vi "EMG_State_Machine.vi"(0 "VISA Refnum in":refnum<visa-resource-name>, 1 "Positions":T4, 2 "EMG signal max amplitude (V)":dbl, 5 "EMG Control":T2(ring), 7 "Mode in":enum16{" M3", " M2", " M1"}(ring), 9 "System calibrated?":bool, 11 "error in (no error)":errorcluster, 12 "New Hand Positions in":T1(array[cluster]), 13 "EMG signal mean amplitude (V)":dbl) -> (3 "Mode":enum16{" M3", " M2", " M1"}(ring), 4 "VISA Refnum out":refnum<visa-resource-name>, 6 "New Hand Positions out":T1(array[cluster]), 8 "Mode out":enum16{" M3", " M2", " M1"}(ring), 10 "Mover4 Data":T3, 15 "error out":errorcluster)   [LabVIEW 2015]
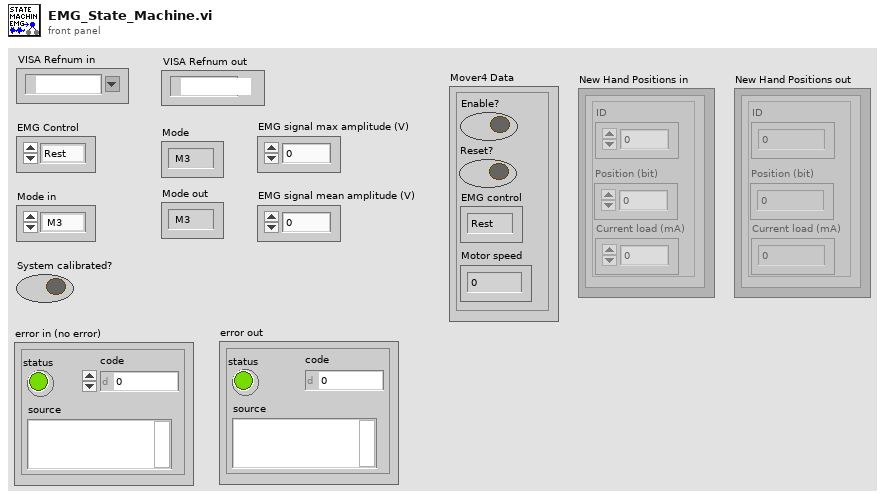
[diagram p1: front panel]
types:
  T1 = cluster{"ID":u16, "Position (bit)":u16, "Current load (mA)":u16}[]
  T2 = enum16{"Rest", "Triceps hardly contracted", "Triceps contracted", "Biceps hardly contracted", "Biceps contracted", "Change mode"}
  T3 = cluster{"Enable?":bool, "Reset?":bool, "EMG control":enum16{"Rest", "Biceps contracted", "Triceps contracted"}, "Motor speed":u8}
  T4 = cluster{"ID":u16, "Position (bit)":u16, "Current load (mA)":u16}
  T5 = enum16{"Rest", "Triceps hardly contracted M3", "Triceps hardly contracted M2", "Triceps hardly contracted M1", "Triceps contracted M3", "Triceps contracted M2", "Triceps contracted M1", "Biceps hardly contracted M3", "Biceps hardly contracted M2", "Biceps hardly contracted M1", "Biceps contracted M3", "Biceps contracted M2", "Biceps contracted M1", "Change mode"}
  T6 = enum16{"Biceps contracted", "Triceps contracted"}
  T7 = enum16{"Biceps contracted M3", "Biceps contracted", "Triceps contracted M3", "Triceps contracted"}
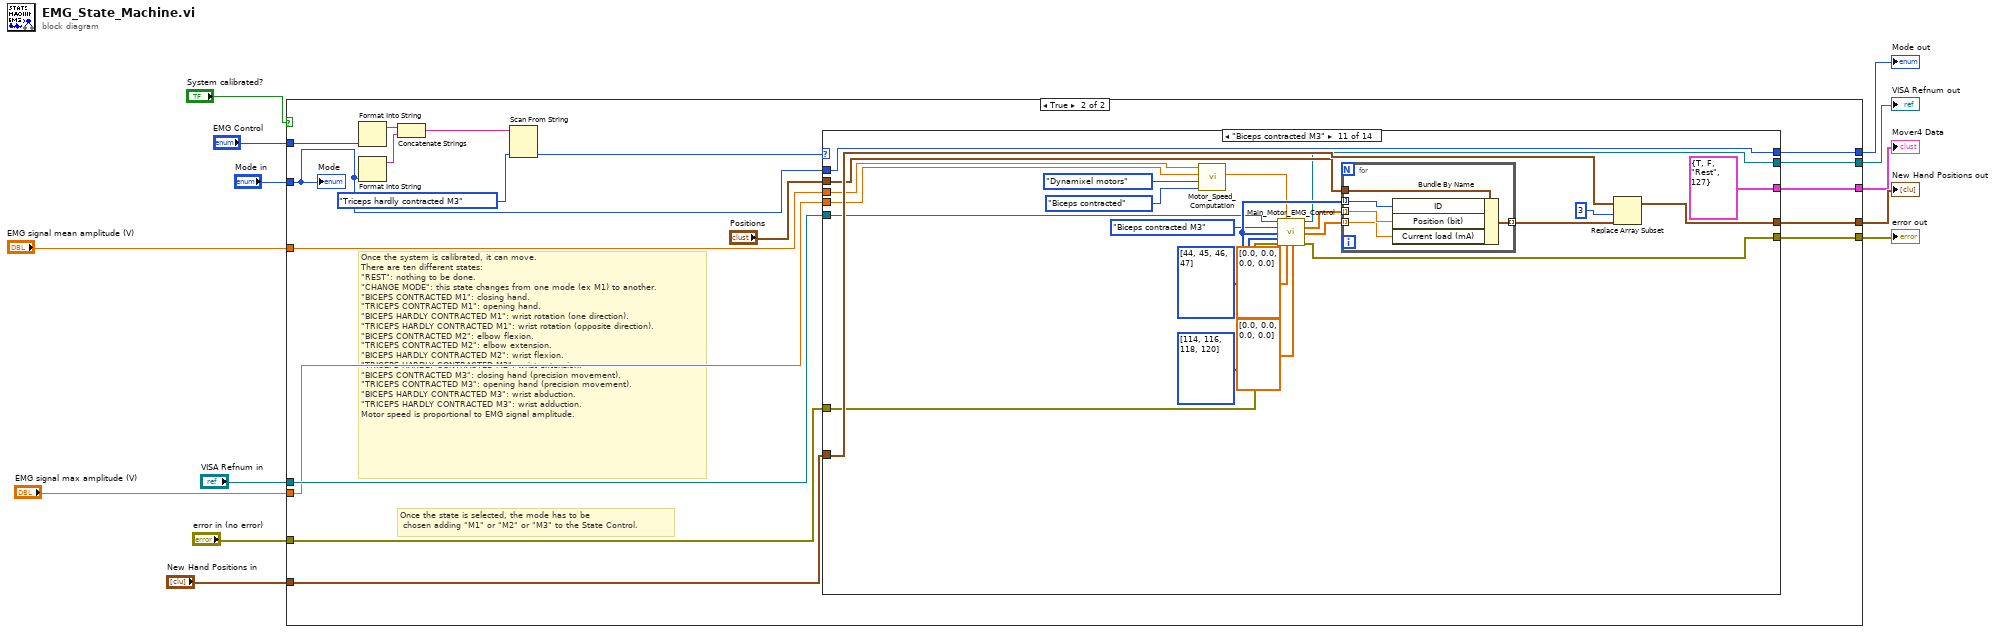
[diagram p0: block diagram]
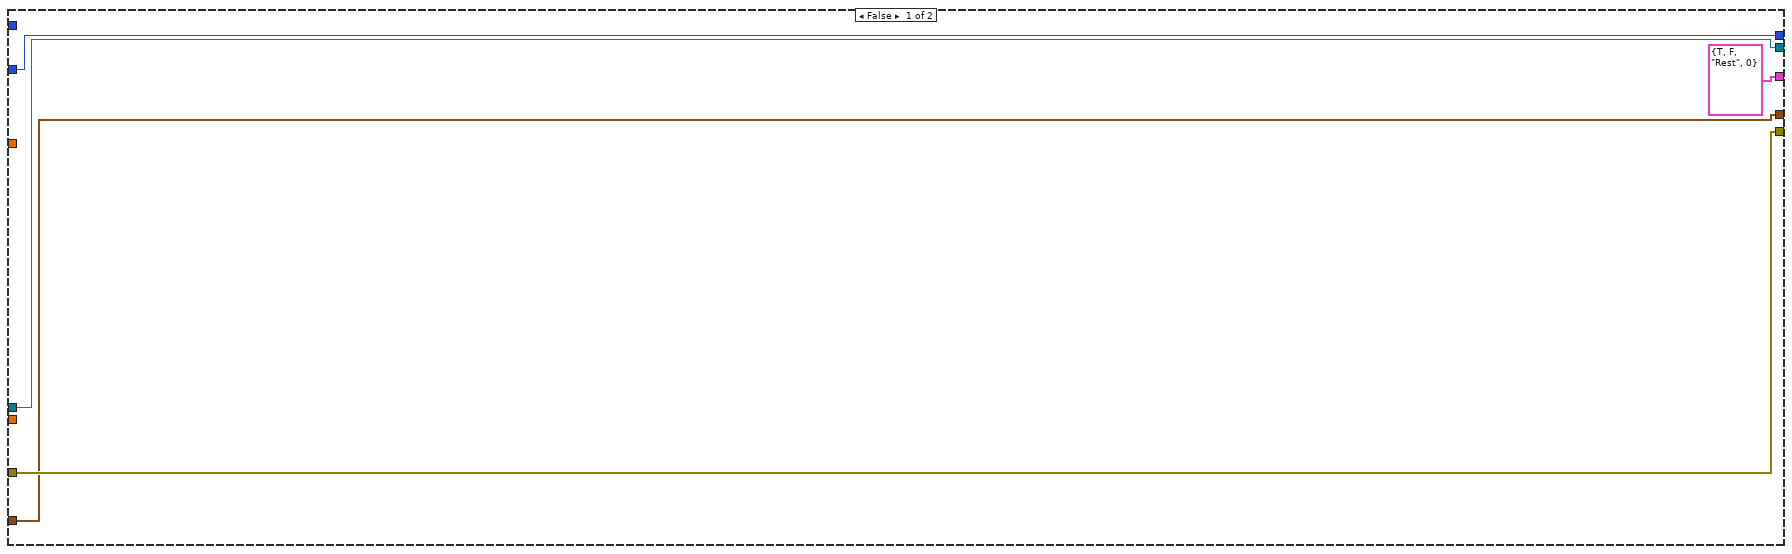
[diagram p2: hidden frame]
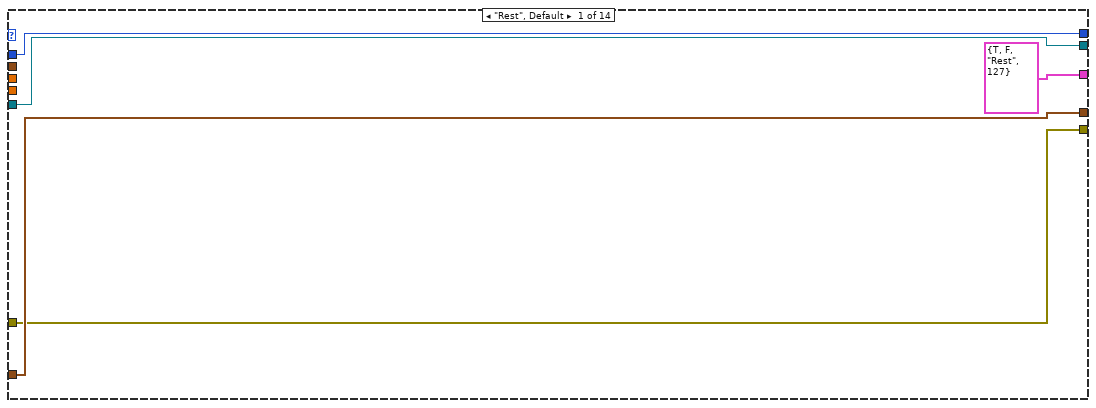
[diagram p3: hidden frame]
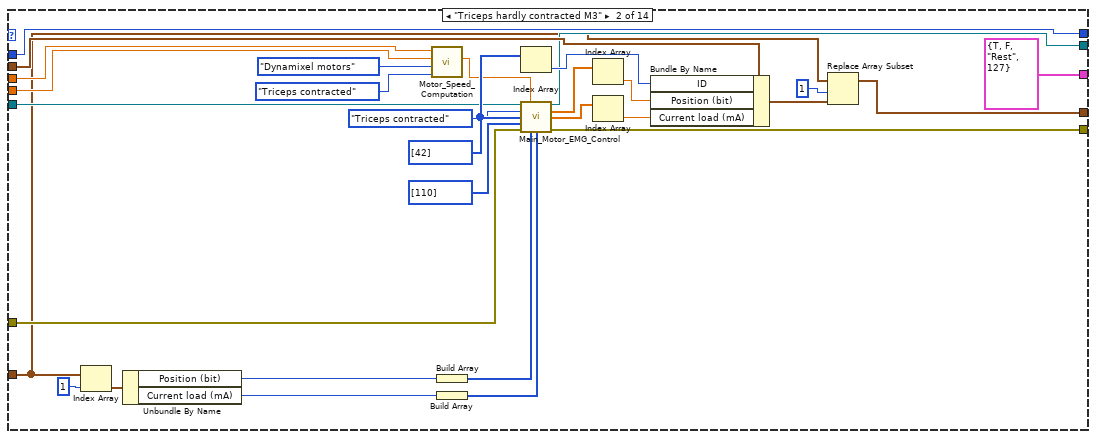
[diagram p4: hidden frame]
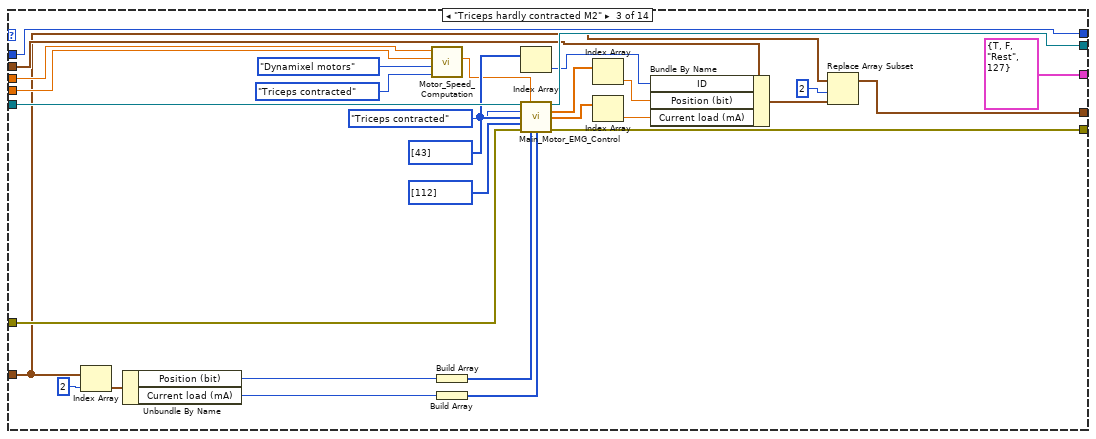
[diagram p5: hidden frame]
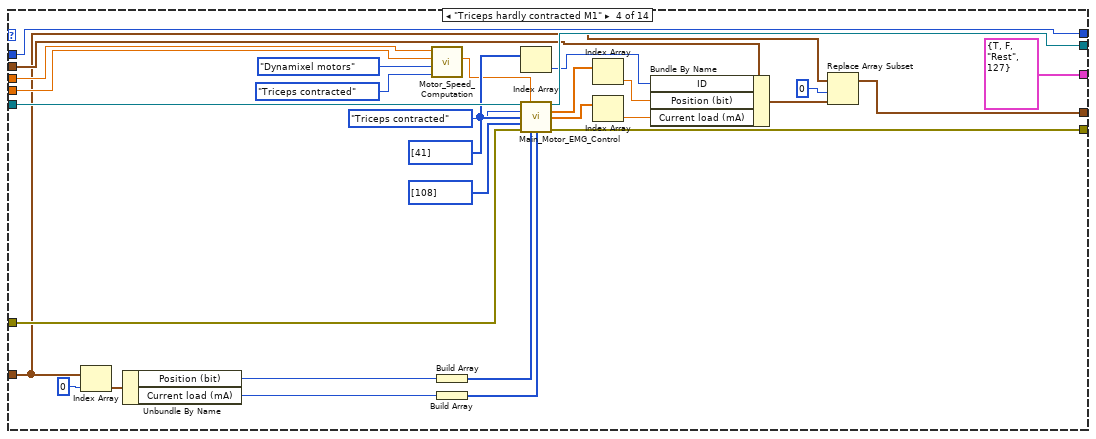
[diagram p6: hidden frame]
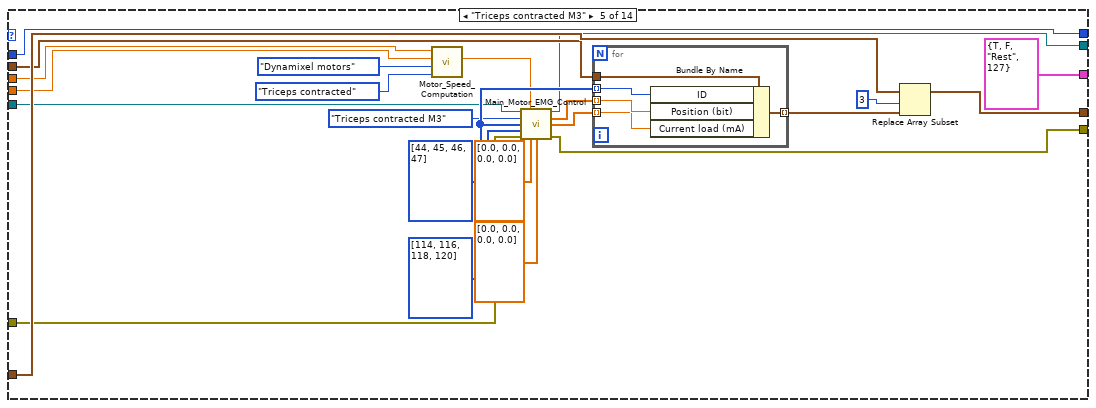
[diagram p7: hidden frame]
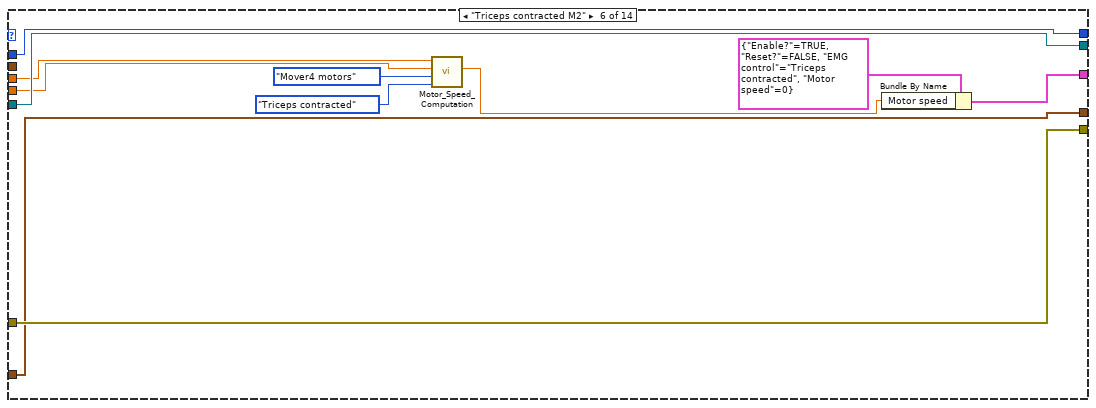
[diagram p8: hidden frame]
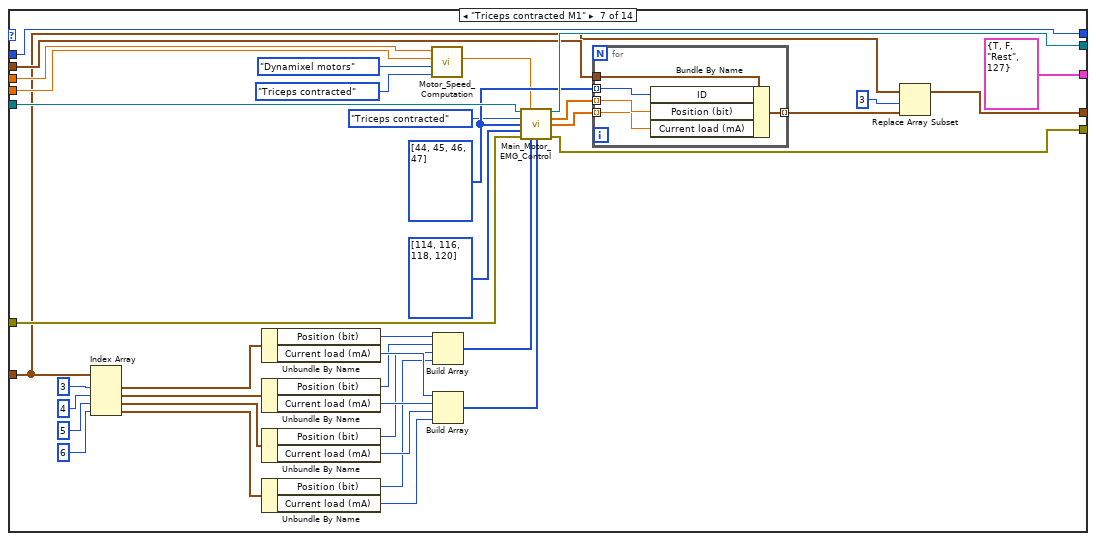
[diagram p9: hidden frame]
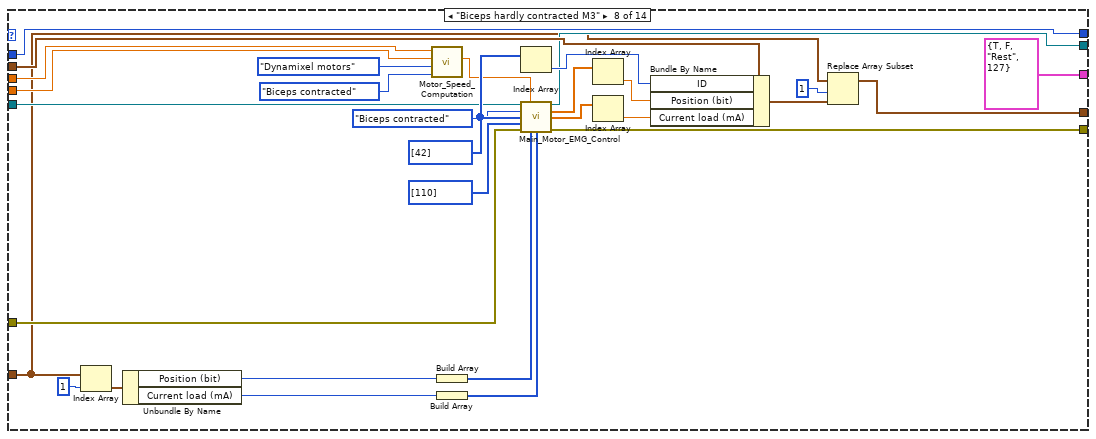
[diagram p10: hidden frame]
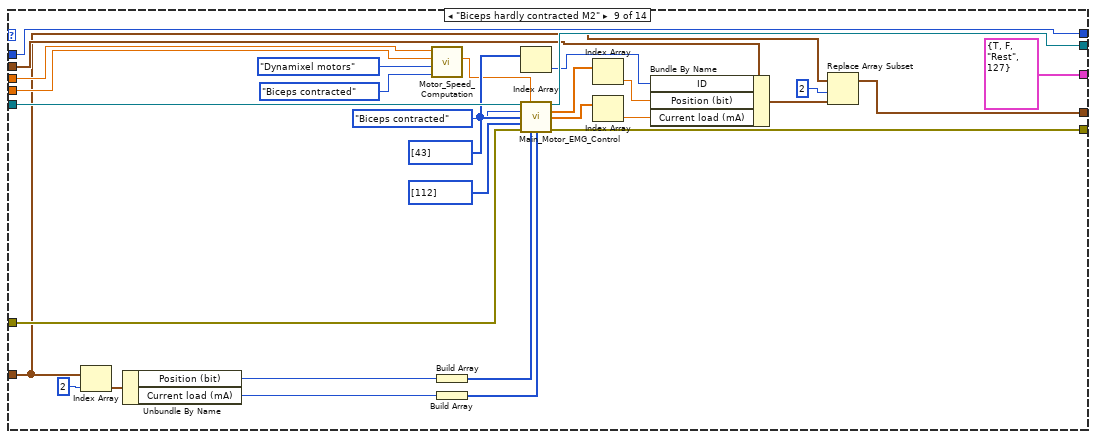
[diagram p11: hidden frame]
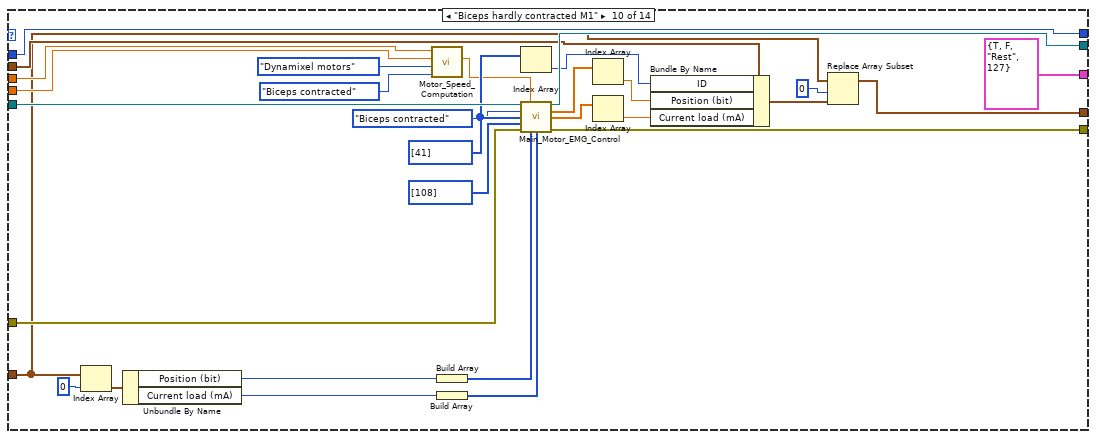
[diagram p12: hidden frame]
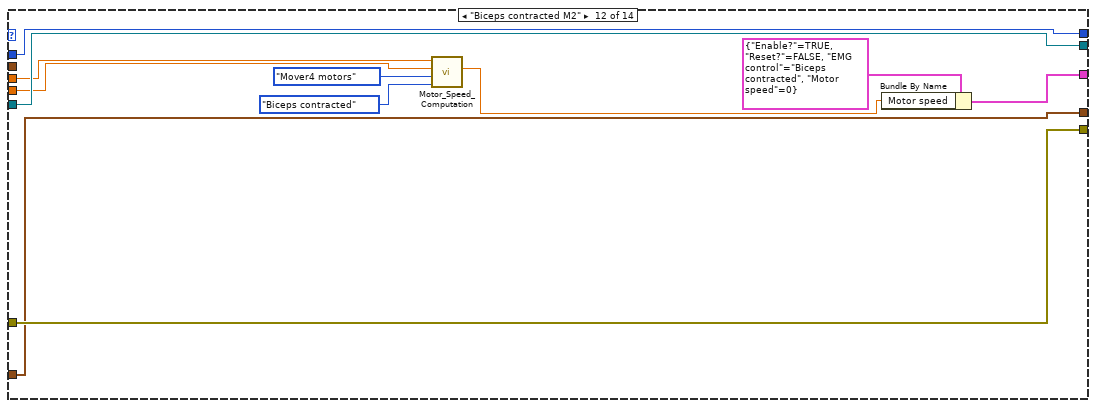
[diagram p13: hidden frame]
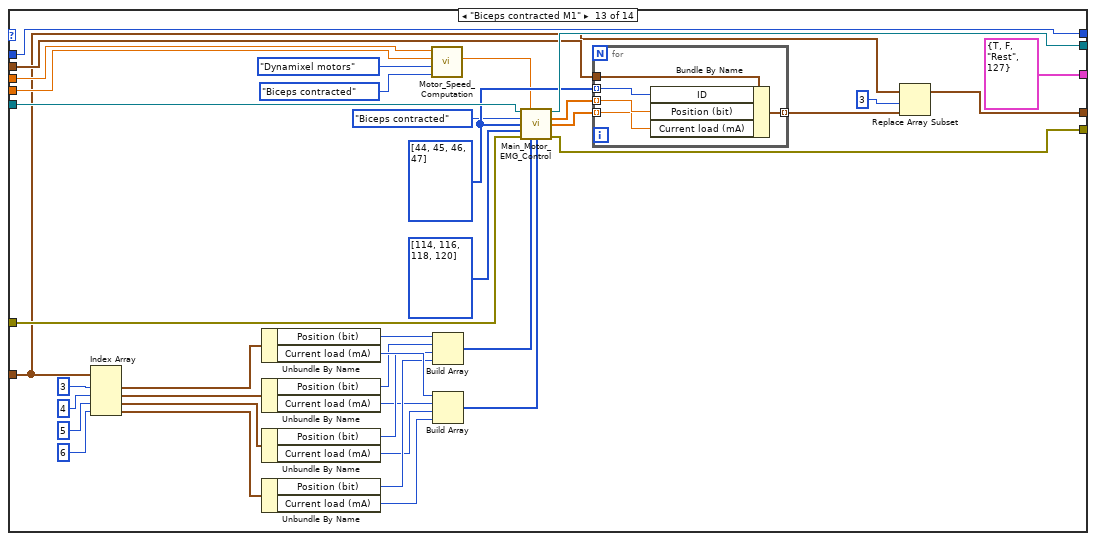
[diagram p14: hidden frame]
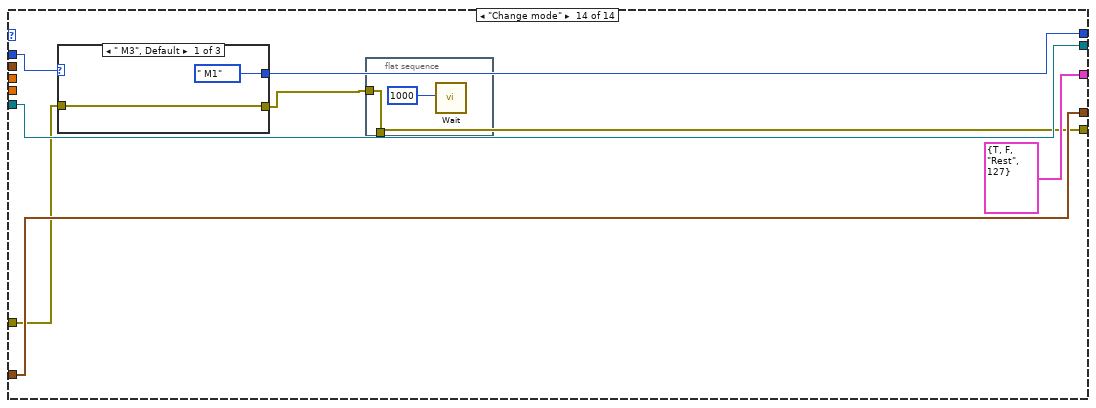
[diagram p15: hidden frame]
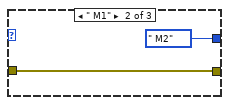
[diagram p16: hidden frame]
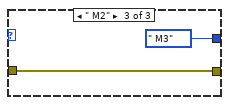
[diagram p17: hidden frame]
diagram:
  n1 = case shown="True" "System calibrated?" {
    tunnel: "VISA Refnum in" -> [w17 w34]
    tunnel: [w15 w23] -> w6
    tunnel: "EMG Control" -> [_ w26]
    tunnel: "error in (no error)" -> [w16 w35]
    tunnel: "Mode in" -> [w18 w27]
    tunnel: [w17 w24] -> w10
    tunnel: [w16 w22] -> w11
    tunnel: [w18 w25] -> w12
    tunnel: "New Hand Positions in" -> [w15 w36]
    tunnel: [T3 {"Enable?"=TRUE, "Reset?"=FALSE, "EMG control"=enum."Rest", "Motor speed"=0} ("data in") w19] -> w1
    tunnel: "EMG signal mean amplitude (V)" -> [_ w21]
    tunnel: "EMG signal max amplitude (V)" -> [_ w20]
    frame False {
    }
    frame True {
      # "Once the state is selected, the mode has to be\n chosen adding \"M1\" or \"M2\" or \"M3\" to the State Control."
      # "Once the system is calibrated, it can move.\nThere are ten different states:\n\"REST\": nothing to be done.\n\"CHANGE MODE\": this state changes from one mode (ex M1) to another.\n\"BICEPS CONTRACTED M1\": closing hand.\n\"TRICEPS CONTRACTED M1\": opening hand.\n\"BICEPS HARDLY CONTRACTED M1\": wrist rotation (one direction).\n\"TRICEPS HARDLY CONTRACTED M1\": wrist rotation (opposite direction).\n\"BICEPS CONTRACTED M2\": elbow flexion.\n\"TRICEPS CONTRACTED M2\": elbow extension.\n\"BICEPS HARDLY CONTRACTED M2\": wrist flexion.\n\"TRICEPS HARDLY CONTRACTED M2\": wrist extension.\n\"BICEPS CONTRACTED M3\": closing hand (precision movement).\n\"TRICEPS CONTRACTED M3\": opening hand (precision movement).\n\"BICEPS HARDLY CONTRACTED M3\": wrist abduction.\n\"TRICEPS HARDLY CONTRACTED M3\": wrist adduction.\nMotor speed is proportional to EMG signal amplitude."
      n2 = Format Into String(w26) -> (resulting string=w32:string)  [unwired: 3 in, 1 out]
      n3 = Format Into String(w27) -> (resulting string=w29:string)  [unwired: 3 in, 1 out]
      n4 = Concatenate Strings(w32, w29) -> (w30:string)
      n5 = Scan From String(input string=w30, default 1=T5."Triceps hardly contracted M3") -> (output 1=w28:T5)  [unwired: 3 in, 3 out]
      n6 = case shown="\"Biceps contracted M3\"" w28 {
        tunnel: w34 -> [w41 w61 w99 w127 w145 w170 w205 w233 w270 w303 w314 w343 w382 w395]
        tunnel: w35 -> [w38 w60 w100 w128 w144 w169 w206 w232 w271 w302 w317 w342 w381 w390]
        tunnel: [w41 w59 w98 w130 w141 w170 w208 w231 w273 w301 w315 w343 w380 w395] -> w24
        tunnel: [w38 w58 w97 w129 w143 w169 w207 w230 w272 w300 w316 w342 w379 w388] -> w22
        tunnel: [w40 w56 w96 w126 w148 w168 w204 w235 w269 w299 w321 w341 w377 w392] -> w25
        tunnel: w27 -> [w40 w56 w96 w126 w148 w168 w204 w235 w269 w299 w321 w341 w377 w393]
        tunnel: w36 -> [w39 w44 w74 w108 w147 w167 w185 w217 w247 w277 w319 w340 w358 w394]
        tunnel: [w39 w57 w87 w120 w142 w167 w199 w229 w264 w294 w320 w340 w374 w394] -> w23
        tunnel: "Positions" -> [_ w62 w86 w116 w146 _ w203 w234 w260 w289 w318 _ w373 _]
        tunnel: [T3 {"Enable?"=TRUE, "Reset?"=FALSE, "EMG control"=enum."Rest", "Motor speed"=127} ("data in") T3 {"Enable?"=TRUE, "Reset?"=FALSE, "EMG control"=enum."Rest", "Motor speed"=127} ("data in") T3 {"Enable?"=TRUE, "Reset?"=FALSE, "EMG control"=enum."Rest", "Motor speed"=127} ("data in") T3 {"Enable?"=TRUE, "Reset?"=FALSE, "EMG control"=enum."Rest", "Motor speed"=127} ("data in") T3 {"Enable?"=TRUE, "Reset?"=FALSE, "EMG control"=enum."Rest", "Motor speed"=127} ("data in") w161 T3 {"Enable?"=TRUE, "Reset?"=FALSE, "EMG control"=enum."Rest", "Motor speed"=127} ("data in") T3 {"Enable?"=TRUE, "Reset?"=FALSE, "EMG control"=enum."Rest", "Motor speed"=127} ("data in") T3 {"Enable?"=TRUE, "Reset?"=FALSE, "EMG control"=enum."Rest", "Motor speed"=127} ("data in") T3 {"Enable?"=TRUE, "Reset?"=FALSE, "EMG control"=enum."Rest", "Motor speed"=127} ("data in") T3 {"Enable?"=TRUE, "Reset?"=FALSE, "EMG control"=enum."Rest", "Motor speed"=127} ("data in") w337 T3 {"Enable?"=TRUE, "Reset?"=FALSE, "EMG control"=enum."Rest", "Motor speed"=127} ("data in") T3 {"Enable?"=TRUE, "Reset?"=FALSE, "EMG control"=enum."Rest", "Motor speed"=127} ("data in")] -> w19
        tunnel: w21 -> [_ w51 w80 w111 w137 w164 w192 w224 w254 w284 w309 w336 w365 _]
        tunnel: w20 -> [_ w50 w81 w112 w136 w163 w191 w223 w253 w283 w308 w335 w366 _]
        frame "Rest", Default {
        }
        frame "Triceps hardly contracted M3" {
          w70 = i32[] [42] ("ID motors")
          n7 = Index Array(array=w44, index=1) -> (element=w47:T4)
          n8 = Unbundle By Name(w47) -> ("Position (bit)"=w46:u16, "Current load (mA)"=w45:u16)
          n9 = call "Motor_Speed_Computation.vi"("Contracted muscle"=T6."Triceps contracted", "Motor type"=enum16{"Mover4 motors", "Dynamixel motors"}."Dynamixel motors", "EMG signal max amplitude (V)"=w50, "EMG signal mean amplitude (V)"=w51) -> ("Motor speed (RPM or bit)"=w52:dbl)  [unwired: 7 in]
          n10 = Build Array(w46) -> (w43:u16[])
          n11 = Build Array(w45) -> (w42:u16[])
          n12 = Index Array(array=w70) -> (element=w69:i32)  [unwired: 1 in]
          n13 = call "Main_Motor_EMG_Control.vi"("VISA Refnum in"=w61, "Motor speed"=w52, "EMG control"=T7."Triceps contracted", "ID motors"=w70, "Address current load"=i32[] [110] ("ID motors"), "error in (no error)"=w60, "Old positions"=w43, "Old Current (mA)"=w42) -> ("VISA Refnum out"=w59:refnum<visa-resource-name>, "Actual positions"=w68:dbl[], "Current (mA)"=w66:dbl[], "error out"=w58:errorcluster)  [unwired: 4 in]
          n14 = Index Array(array=w68) -> (element=w67:dbl)  [unwired: 1 in]
          n15 = Index Array(array=w66) -> (element=w65:dbl)  [unwired: 1 in]
          n16 = Bundle By Name(cluster=w62, "ID"=w69, "Position (bit)"=w67, "Current load (mA)"=w65) -> (w64:T4)
          n17 = Replace Array Subset(array=w44, new element=w64, index=1) -> (w57:T1)
        }
        frame "Triceps hardly contracted M2" {
          w95 = i32[] [43] ("ID motors")
          n18 = Index Array(array=w74, index=2) -> (element=w77:T4)
          n19 = Unbundle By Name(w77) -> ("Position (bit)"=w76:u16, "Current load (mA)"=w75:u16)
          n20 = call "Motor_Speed_Computation.vi"("Contracted muscle"=T6."Triceps contracted", "Motor type"=enum16{"Mover4 motors", "Dynamixel motors"}."Dynamixel motors", "EMG signal max amplitude (V)"=w81, "EMG signal mean amplitude (V)"=w80) -> ("Motor speed (RPM or bit)"=w82:dbl)  [unwired: 7 in]
          n21 = Build Array(w76) -> (w73:u16[])
          n22 = Build Array(w75) -> (w72:u16[])
          n23 = Index Array(array=w95) -> (element=w94:i32)  [unwired: 1 in]
          n24 = call "Main_Motor_EMG_Control.vi"("VISA Refnum in"=w99, "Motor speed"=w82, "EMG control"=T7."Triceps contracted", "ID motors"=w95, "Address current load"=i32[] [112] ("ID motors"), "error in (no error)"=w100, "Old positions"=w73, "Old Current (mA)"=w72) -> ("VISA Refnum out"=w98:refnum<visa-resource-name>, "Actual positions"=w93:dbl[], "Current (mA)"=w91:dbl[], "error out"=w97:errorcluster)  [unwired: 4 in]
          n25 = Index Array(array=w93) -> (element=w92:dbl)  [unwired: 1 in]
          n26 = Index Array(array=w91) -> (element=w90:dbl)  [unwired: 1 in]
          n27 = Bundle By Name(cluster=w86, "ID"=w94, "Position (bit)"=w92, "Current load (mA)"=w90) -> (w89:T4)
          n28 = Replace Array Subset(array=w74, new element=w89, index=2) -> (w87:T1)
        }
        frame "Triceps hardly contracted M1" {
          w119 = i32[] [41] ("ID motors")
          n29 = Index Array(array=w108, index=0) -> (element=w106:T4)
          n30 = Unbundle By Name(w106) -> ("Position (bit)"=w105:u16, "Current load (mA)"=w103:u16)
          n31 = call "Motor_Speed_Computation.vi"("Contracted muscle"=T6."Triceps contracted", "Motor type"=enum16{"Mover4 motors", "Dynamixel motors"}."Dynamixel motors", "EMG signal max amplitude (V)"=w112, "EMG signal mean amplitude (V)"=w111) -> ("Motor speed (RPM or bit)"=w110:dbl)  [unwired: 7 in]
          n32 = Build Array(w105) -> (w104:u16[])
          n33 = Build Array(w103) -> (w102:u16[])
          n34 = Index Array(array=w119) -> (element=w125:i32)  [unwired: 1 in]
          n35 = call "Main_Motor_EMG_Control.vi"("VISA Refnum in"=w127, "Motor speed"=w110, "EMG control"=T7."Triceps contracted", "ID motors"=w119, "Address current load"=i32[] [108] ("ID motors"), "error in (no error)"=w128, "Old positions"=w104, "Old Current (mA)"=w102) -> ("VISA Refnum out"=w130:refnum<visa-resource-name>, "Actual positions"=w118:dbl[], "Current (mA)"=w117:dbl[], "error out"=w129:errorcluster)  [unwired: 4 in]
          n36 = Index Array(array=w118) -> (element=w124:dbl)  [unwired: 1 in]
          n37 = Index Array(array=w117) -> (element=w123:dbl)  [unwired: 1 in]
          n38 = Bundle By Name(cluster=w116, "ID"=w125, "Position (bit)"=w124, "Current load (mA)"=w123) -> (w122:T4)
          n39 = Replace Array Subset(array=w108, new element=w122, index=0) -> (w120:T1)
        }
        frame "Triceps contracted M3" {
          w151 = i32[] [44, 45, 46, 47] ("ID motors")
          n40 = call "Motor_Speed_Computation.vi"("Contracted muscle"=T6."Triceps contracted", "Motor type"=enum16{"Mover4 motors", "Dynamixel motors"}."Dynamixel motors", "EMG signal max amplitude (V)"=w136, "EMG signal mean amplitude (V)"=w137) -> ("Motor speed (RPM or bit)"=w135:dbl)  [unwired: 7 in]
          n41 = call "Main_Motor_EMG_Control.vi"("VISA Refnum in"=w145, "Motor speed"=w135, "EMG control"=T7."Triceps contracted M3", "ID motors"=w151, "Address current load"=i32[] [114, 116, 118, 120] ("ID motors"), "error in (no error)"=w144, "Old positions"=dbl[] [0.0, 0.0, 0.0, 0.0], "Old Current (mA)"=dbl[] [0.0, 0.0, 0.0, 0.0]) -> ("VISA Refnum out"=w141:refnum<visa-resource-name>, "Actual positions"=w150:dbl[], "Current (mA)"=w149:dbl[], "error out"=w143:errorcluster)  [unwired: 4 in]
          n42 = for {
            tunnel: w146 -> [w159]
            tunnel: w151 -> [w158] mode=indexing
            tunnel: w150 -> [w157] mode=indexing
            tunnel: w149 -> [w156] mode=indexing
            tunnel: [w155] -> w153 mode=indexing
            n43 = Bundle By Name(cluster=w159, "ID"=w158, "Position (bit)"=w157, "Current load (mA)"=w156) -> (w155:T4)
          }
          n44 = Replace Array Subset(array=w147, new element=w153, index=3) -> (w142:T1)
        }
        frame "Triceps contracted M2" {
          n45 = call "Motor_Speed_Computation.vi"("Contracted muscle"=T6."Triceps contracted", "Motor type"=enum16{"Mover4 motors", "Dynamixel motors"}."Mover4 motors", "EMG signal max amplitude (V)"=w163, "EMG signal mean amplitude (V)"=w164) -> ("Motor speed (RPM or bit)"=w162:dbl)  [unwired: 7 in]
          n46 = Bundle By Name(cluster=T3 {"Enable?"=TRUE, "Reset?"=FALSE, "EMG control"=enum."Triceps contracted", "Motor speed"=0} ("data in"), "Motor speed"=w162) -> (w161:T3)
        }
        frame "Triceps contracted M1" {
          w202 = i32[] [44, 45, 46, 47] ("ID motors")
          n47 = Index Array(array=w185, index #1=3 ("index"), index #2=4 ("index"), index #3=5 ("index"), index #4=6 ("index")) -> (element #1=w188:T4, element #2=w179:T4, element #3=w178:T4, element #4=w177:T4)
          n48 = Unbundle By Name(w188) -> ("Position (bit)"=w187:u16, "Current load (mA)"=w186:u16)
          n49 = Unbundle By Name(w179) -> ("Position (bit)"=w173:u16, "Current load (mA)"=w176:u16)
          n50 = Unbundle By Name(w178) -> ("Position (bit)"=w172:u16, "Current load (mA)"=w175:u16)
          n51 = Unbundle By Name(w177) -> ("Position (bit)"=w171:u16, "Current load (mA)"=w174:u16)
          n52 = call "Motor_Speed_Computation.vi"("Contracted muscle"=T6."Triceps contracted", "Motor type"=enum16{"Mover4 motors", "Dynamixel motors"}."Dynamixel motors", "EMG signal max amplitude (V)"=w191, "EMG signal mean amplitude (V)"=w192) -> ("Motor speed (RPM or bit)"=w190:dbl)  [unwired: 7 in]
          n53 = Build Array(w187, w173, w172, w171) -> (w181:u16[])
          n54 = Build Array(w186, w176, w175, w174) -> (w180:u16[])
          n55 = call "Main_Motor_EMG_Control.vi"("VISA Refnum in"=w205, "Motor speed"=w190, "EMG control"=T7."Triceps contracted", "ID motors"=w202, "Address current load"=i32[] [114, 116, 118, 120] ("ID motors"), "error in (no error)"=w206, "Old positions"=w181, "Old Current (mA)"=w180) -> ("VISA Refnum out"=w208:refnum<visa-resource-name>, "Actual positions"=w201:dbl[], "Current (mA)"=w200:dbl[], "error out"=w207:errorcluster)  [unwired: 4 in]
          n56 = for {
            tunnel: w203 -> [w214]
            tunnel: w202 -> [w213] mode=indexing
            tunnel: w201 -> [w212] mode=indexing
            tunnel: w200 -> [w211] mode=indexing
            tunnel: [w210] -> w198 mode=indexing
            n57 = Bundle By Name(cluster=w214, "ID"=w213, "Position (bit)"=w212, "Current load (mA)"=w211) -> (w210:T4)
          }
          n58 = Replace Array Subset(array=w185, new element=w198, index=3) -> (w199:T1)
        }
        frame "Biceps hardly contracted M3" {
          w243 = i32[] [42] ("ID motors")
          n59 = Index Array(array=w217, index=1) -> (element=w220:T4)
          n60 = Unbundle By Name(w220) -> ("Position (bit)"=w219:u16, "Current load (mA)"=w218:u16)
          n61 = call "Motor_Speed_Computation.vi"("Contracted muscle"=T6."Biceps contracted", "Motor type"=enum16{"Mover4 motors", "Dynamixel motors"}."Dynamixel motors", "EMG signal max amplitude (V)"=w223, "EMG signal mean amplitude (V)"=w224) -> ("Motor speed (RPM or bit)"=w222:dbl)  [unwired: 7 in]
          n62 = Build Array(w219) -> (w216:u16[])
          n63 = Build Array(w218) -> (w215:u16[])
          n64 = Index Array(array=w243) -> (element=w242:i32)  [unwired: 1 in]
          n65 = call "Main_Motor_EMG_Control.vi"("VISA Refnum in"=w233, "Motor speed"=w222, "EMG control"=T7."Biceps contracted", "ID motors"=w243, "Address current load"=i32[] [110] ("ID motors"), "error in (no error)"=w232, "Old positions"=w216, "Old Current (mA)"=w215) -> ("VISA Refnum out"=w231:refnum<visa-resource-name>, "Actual positions"=w241:dbl[], "Current (mA)"=w239:dbl[], "error out"=w230:errorcluster)  [unwired: 4 in]
          n66 = Index Array(array=w241) -> (element=w240:dbl)  [unwired: 1 in]
          n67 = Index Array(array=w239) -> (element=w238:dbl)  [unwired: 1 in]
          n68 = Bundle By Name(cluster=w234, "ID"=w242, "Position (bit)"=w240, "Current load (mA)"=w238) -> (w237:T4)
          n69 = Replace Array Subset(array=w217, new element=w237, index=1) -> (w229:T1)
        }
        frame "Biceps hardly contracted M2" {
          w263 = i32[] [43] ("ID motors")
          n70 = Index Array(array=w247, index=2) -> (element=w250:T4)
          n71 = Unbundle By Name(w250) -> ("Position (bit)"=w249:u16, "Current load (mA)"=w248:u16)
          n72 = call "Motor_Speed_Computation.vi"("Contracted muscle"=T6."Biceps contracted", "Motor type"=enum16{"Mover4 motors", "Dynamixel motors"}."Dynamixel motors", "EMG signal max amplitude (V)"=w253, "EMG signal mean amplitude (V)"=w254) -> ("Motor speed (RPM or bit)"=w252:dbl)  [unwired: 7 in]
          n73 = Build Array(w249) -> (w246:u16[])
          n74 = Build Array(w248) -> (w245:u16[])
          n75 = Index Array(array=w263) -> (element=w268:i32)  [unwired: 1 in]
          n76 = call "Main_Motor_EMG_Control.vi"("VISA Refnum in"=w270, "Motor speed"=w252, "EMG control"=T7."Biceps contracted", "ID motors"=w263, "Address current load"=i32[] [112] ("ID motors"), "error in (no error)"=w271, "Old positions"=w246, "Old Current (mA)"=w245) -> ("VISA Refnum out"=w273:refnum<visa-resource-name>, "Actual positions"=w262:dbl[], "Current (mA)"=w261:dbl[], "error out"=w272:errorcluster)  [unwired: 4 in]
          n77 = Index Array(array=w262) -> (element=w267:dbl)  [unwired: 1 in]
          n78 = Index Array(array=w261) -> (element=w259:dbl)  [unwired: 1 in]
          n79 = Bundle By Name(cluster=w260, "ID"=w268, "Position (bit)"=w267, "Current load (mA)"=w259) -> (w266:T4)
          n80 = Replace Array Subset(array=w247, new element=w266, index=2) -> (w264:T1)
        }
        frame "Biceps hardly contracted M1" {
          w293 = i32[] [41] ("ID motors")
          n81 = Index Array(array=w277, index=0) -> (element=w280:T4)
          n82 = Unbundle By Name(w280) -> ("Position (bit)"=w279:u16, "Current load (mA)"=w278:u16)
          n83 = call "Motor_Speed_Computation.vi"("Contracted muscle"=T6."Biceps contracted", "Motor type"=enum16{"Mover4 motors", "Dynamixel motors"}."Dynamixel motors", "EMG signal max amplitude (V)"=w283, "EMG signal mean amplitude (V)"=w284) -> ("Motor speed (RPM or bit)"=w282:dbl)  [unwired: 7 in]
          n84 = Build Array(w279) -> (w276:u16[])
          n85 = Build Array(w278) -> (w275:u16[])
          n86 = Index Array(array=w293) -> (element=w298:i32)  [unwired: 1 in]
          n87 = call "Main_Motor_EMG_Control.vi"("VISA Refnum in"=w303, "Motor speed"=w282, "EMG control"=T7."Biceps contracted", "ID motors"=w293, "Address current load"=i32[] [108] ("ID motors"), "error in (no error)"=w302, "Old positions"=w276, "Old Current (mA)"=w275) -> ("VISA Refnum out"=w301:refnum<visa-resource-name>, "Actual positions"=w292:dbl[], "Current (mA)"=w291:dbl[], "error out"=w300:errorcluster)  [unwired: 4 in]
          n88 = Index Array(array=w292) -> (element=w297:dbl)  [unwired: 1 in]
          n89 = Index Array(array=w291) -> (element=w290:dbl)  [unwired: 1 in]
          n90 = Bundle By Name(cluster=w289, "ID"=w298, "Position (bit)"=w297, "Current load (mA)"=w290) -> (w296:T4)
          n91 = Replace Array Subset(array=w277, new element=w296, index=0) -> (w294:T1)
        }
        frame "Biceps contracted M3" {
          w324 = i32[] [44, 45, 46, 47] ("ID motors")
          n92 = call "Motor_Speed_Computation.vi"("Contracted muscle"=T6."Biceps contracted", "Motor type"=enum16{"Mover4 motors", "Dynamixel motors"}."Dynamixel motors", "EMG signal max amplitude (V)"=w308, "EMG signal mean amplitude (V)"=w309) -> ("Motor speed (RPM or bit)"=w307:dbl)  [unwired: 7 in]
          n93 = call "Main_Motor_EMG_Control.vi"("VISA Refnum in"=w314, "Motor speed"=w307, "EMG control"=T7."Biceps contracted M3", "ID motors"=w324, "Address current load"=i32[] [114, 116, 118, 120] ("ID motors"), "error in (no error)"=w317, "Old positions"=dbl[] [0.0, 0.0, 0.0, 0.0], "Old Current (mA)"=dbl[] [0.0, 0.0, 0.0, 0.0]) -> ("VISA Refnum out"=w315:refnum<visa-resource-name>, "Actual positions"=w323:dbl[], "Current (mA)"=w322:dbl[], "error out"=w316:errorcluster)  [unwired: 4 in]
          n94 = for {
            tunnel: w318 -> [w332]
            tunnel: w324 -> [w331] mode=indexing
            tunnel: w323 -> [w330] mode=indexing
            tunnel: w322 -> [w329] mode=indexing
            tunnel: [w328] -> w326 mode=indexing
            n95 = Bundle By Name(cluster=w332, "ID"=w331, "Position (bit)"=w330, "Current load (mA)"=w329) -> (w328:T4)
          }
          n96 = Replace Array Subset(array=w319, new element=w326, index=3) -> (w320:T1)
        }
        frame "Biceps contracted M2" {
          n97 = call "Motor_Speed_Computation.vi"("Contracted muscle"=T6."Biceps contracted", "Motor type"=enum16{"Mover4 motors", "Dynamixel motors"}."Mover4 motors", "EMG signal max amplitude (V)"=w335, "EMG signal mean amplitude (V)"=w336) -> ("Motor speed (RPM or bit)"=w339:dbl)  [unwired: 7 in]
          n98 = Bundle By Name(cluster=T3 {"Enable?"=TRUE, "Reset?"=FALSE, "EMG control"=enum."Biceps contracted", "Motor speed"=0} ("data in"), "Motor speed"=w339) -> (w337:T3)
        }
        frame "Biceps contracted M1" {
          w372 = i32[] [44, 45, 46, 47] ("ID motors")
          n99 = Index Array(array=w358, index #1=3 ("index"), index #2=4 ("index"), index #3=5 ("index"), index #4=6 ("index")) -> (element #1=w361:T4, element #2=w354:T4, element #3=w353:T4, element #4=w352:T4)
          n100 = Unbundle By Name(w361) -> ("Position (bit)"=w360:u16, "Current load (mA)"=w359:u16)
          n101 = Unbundle By Name(w354) -> ("Position (bit)"=w351:u16, "Current load (mA)"=w347:u16)
          n102 = Unbundle By Name(w353) -> ("Position (bit)"=w350:u16, "Current load (mA)"=w346:u16)
          n103 = Unbundle By Name(w352) -> ("Position (bit)"=w349:u16, "Current load (mA)"=w345:u16)
          n104 = call "Motor_Speed_Computation.vi"("Contracted muscle"=T6."Biceps contracted", "Motor type"=enum16{"Mover4 motors", "Dynamixel motors"}."Dynamixel motors", "EMG signal max amplitude (V)"=w366, "EMG signal mean amplitude (V)"=w365) -> ("Motor speed (RPM or bit)"=w364:dbl)  [unwired: 7 in]
          n105 = Build Array(w360, w351, w350, w349) -> (w348:u16[])
          n106 = Build Array(w359, w347, w346, w345) -> (w344:u16[])
          n107 = call "Main_Motor_EMG_Control.vi"("VISA Refnum in"=w382, "Motor speed"=w364, "EMG control"=T7."Biceps contracted", "ID motors"=w372, "Address current load"=i32[] [114, 116, 118, 120] ("ID motors"), "error in (no error)"=w381, "Old positions"=w348, "Old Current (mA)"=w344) -> ("VISA Refnum out"=w380:refnum<visa-resource-name>, "Actual positions"=w371:dbl[], "Current (mA)"=w370:dbl[], "error out"=w379:errorcluster)  [unwired: 4 in]
          n108 = for {
            tunnel: w373 -> [w387]
            tunnel: w372 -> [w386] mode=indexing
            tunnel: w371 -> [w385] mode=indexing
            tunnel: w370 -> [w384] mode=indexing
            tunnel: [w383] -> w376 mode=indexing
            n109 = Bundle By Name(cluster=w387, "ID"=w386, "Position (bit)"=w385, "Current load (mA)"=w384) -> (w383:T4)
          }
          n110 = Replace Array Subset(array=w358, new element=w376, index=3) -> (w374:T1)
        }
        frame "Change mode" {
          n111 = case shown="\" M3\", Default" w393 {
            tunnel: [enum16{" M3", " M2", " M1"}." M1" ("Mode Out") enum16{" M3", " M2", " M1"}." M2" ("Mode Out") enum16{" M3", " M2", " M1"}." M3" ("Mode Out")] -> w392
            tunnel: w390 -> [w398 w400 w402]
            tunnel: [w398 w400 w402] -> w389
            frame " M3", Default {
            }
            frame " M1" {
            }
            frame " M2" {
            }
          }
          n112 = flat-sequence {
            tunnel: w389 -> [w397]
            tunnel: [w397] -> w388
            frame #0 {
              n113 = call "Wait"("Count(mSec)"=u32 1000 ("Tick Count(mSec)")) -> ()  [unwired: 1 out]
            }
          }
        }
      }
      "Mode" <- w27
    }
  }
  "Mover4 Data" <- w1
  "Mode out" <- w12
  "error out" <- w11
  "VISA Refnum out" <- w10
  "New Hand Positions out" <- w6
